vi "GetAutoGainHeight.vi"(8 "错误输入（无错误）":errorcluster) -> (0 "错误输出":errorcluster, 3 "自动增益波高百分比":u16)   [LabVIEW 2014]
uses:
  X86Dll/ZXUTConfigMgr.dll
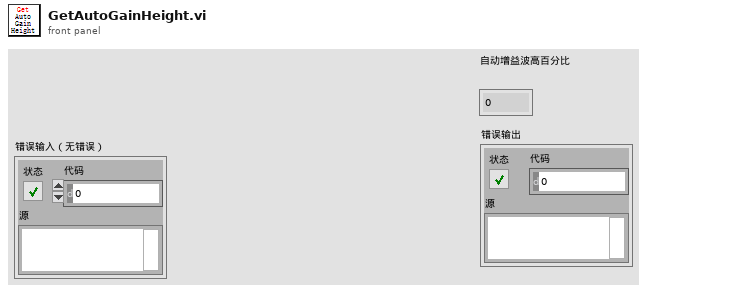
[diagram p1: front panel]
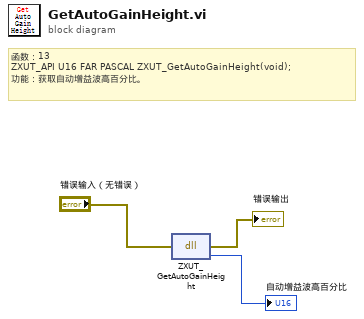
[diagram p0: block diagram]
diagram:
  # "函数：13\nZXUT_API U16\tFAR PASCAL ZXUT_GetAutoGainHeight(void);\n功能：获取自动增益波高百分比。"
  n1 = dll-call lib="D:/Software/Utrasonic on-line monitoring/X86Dll/ZXUTConfigMgr.dll" fn="ZXUT_GetAutoGainHeight"(error in="错误输入（无错误）") -> (error out=→"错误输出":errorcluster, "返回类型"=→"自动增益波高百分比":u16)  [unwired: 2 in, 1 out]
